vi "GetProperties.vi"(8 "error in":errorcluster, 11 "NumericWithScale in":refnum<class "NumericWithScale.lvclass">) -> (0 "error out":errorcluster, 3 "NumericWithScale out":refnum<class "NumericWithScale.lvclass">)   [LabVIEW 2014, in "NumericWithScale.lvclass"]
uses:
  NumericWithScale.lvclass
  NumericWithScale.lvclass/NumericWithScale.ctl
  Numeric/Numeric.lvclass
  Digital/Digital.lvclass
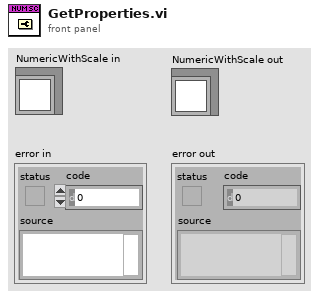
[diagram p1: front panel]
types:
  T1 = typedef "LVForegroundBackgroundColorsTypeDef.ctl" = cluster{"FG Color":u32, "BG Color":u32}
  T2 = typedef "LVBoundsTypeDef.ctl" = cluster{"Width":u32, "Height":u32}
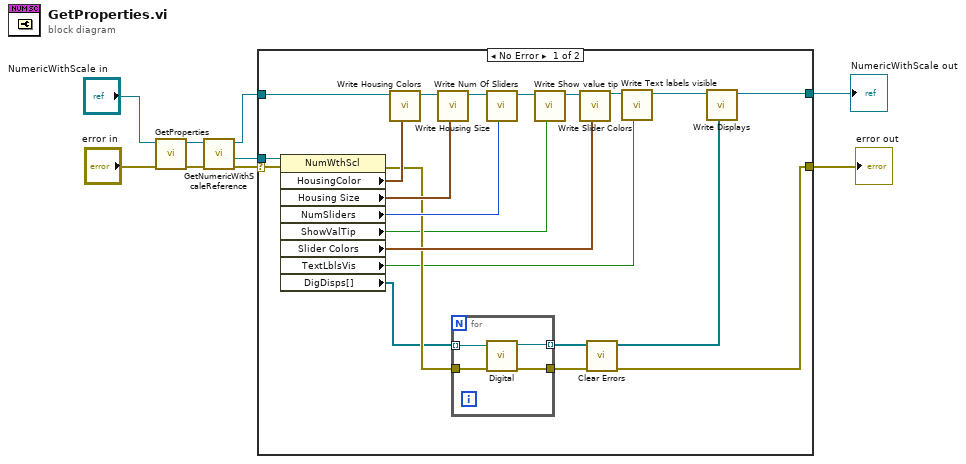
[diagram p0: block diagram]
diagram:
  n1 = call-parent "GetProperties.vi"("error in"="error in", "Numeric in"="NumericWithScale in") -> ("error out"=w6:errorcluster, "Numeric out"=w7:refnum<class "NumericWithScale.lvclass">)  [unwired: 8 in]
  n2 = call "GetNumericWithScaleReference.vi"("error in"=w6, "NumericWithScale in"=w7) -> ("error out"=w5:errorcluster, "numeric with scale reference"=w4:refnum<vi>, "NumericWithScale out"=w3:refnum<class "NumericWithScale.lvclass">)  [unwired: 7 in]
  n3 = case shown="No Error" w5 {
    selector: w5 -> [w29 w36]
    tunnel: w4 -> [w30 _]
    tunnel: w3 -> [w28 w35]
    tunnel: [w19 w35] -> w2
    tunnel: [w10 w36] -> w1
    frame No Error {
      n4 = property class="NumWthScl"(reference=w30, error in=w29) -> (error out=w21:errorcluster, "HousingColor"=w27:T1, "Housing Size"=w25:T2, "NumSliders"=w23:i32, "ShowValTip"=w13:bool, "Slider Colors"=w22:T1, "TextLblsVis"=w16:bool, "DigDisps[]"=w12:refnum<vi>[])  [unwired: 1 out]
      n5 = call "Write Housing Colors.vi"("Housing Colors"=w27, "NumericWithScale in"=w28) -> ("NumericWithScale out"=w26:refnum<class "NumericWithScale.lvclass">)  [unwired: 7 in]
      n6 = call "Write Housing Size.vi"("Housing Size"=w25, "NumericWithScale in"=w26) -> ("NumericWithScale out"=w24:refnum<class "NumericWithScale.lvclass">)  [unwired: 7 in]
      n7 = for {
        tunnel: w12 -> [w33] mode=indexing
        tunnel: [w31] -> w20 mode=indexing
        tunnel: w21 -> [w34]
        tunnel: [w32] -> w18
        n8 = call "Digital.vi"("error in"=w34, "GObj Refnum"=w33) -> ("error out"=w32:errorcluster, "Digital out"=w31:refnum<class "Digital.lvclass">)  [unwired: 8 in]
      }
      n9 = call "Write Num Of Sliders.vi"("Num Of Sliders"=w23, "NumericWithScale in"=w24) -> ("NumericWithScale out"=w15:refnum<class "NumericWithScale.lvclass">)  [unwired: 7 in]
      n10 = call "Write Show value tip.vi"("Show value tip"=w13, "NumericWithScale in"=w15) -> ("NumericWithScale out"=w14:refnum<class "NumericWithScale.lvclass">)  [unwired: 7 in]
      n11 = call "Write Slider Colors.vi"("Slider Colors"=w22, "NumericWithScale in"=w14) -> ("NumericWithScale out"=w17:refnum<class "NumericWithScale.lvclass">)  [unwired: 7 in]
      n12 = call <vilib>:"Clear Errors.vi"("error in (no error)"=w18) -> ("error out"=w10:errorcluster)  [unwired: 5 in, 1 out]
      n13 = call "Write Text labels visible.vi"("Text labels visible"=w16, "NumericWithScale in"=w17) -> ("NumericWithScale out"=w11:refnum<class "NumericWithScale.lvclass">)  [unwired: 7 in]
      n14 = call "Write Displays.vi"("Displays"=w20, "NumericWithScale in"=w11) -> ("NumericWithScale out"=w19:refnum<class "NumericWithScale.lvclass">)  [unwired: 7 in]
    }
    frame Error {
    }
  }
  "error out" <- w1
  "NumericWithScale out" <- w2
